vi "(SubVI) path to xy data.vi"(10 "base path":path, 11 "name or relative path":string) -> (1 "all y position\n(pixel)":dbl[][](array[numeric]), 2 "all x position\n(pixel)":dbl[][](array[numeric]), 3 "Tandem Yi position":dbl[](array[numeric]), 4 "# of frames":dbl, 5 "Tandem Xi position":dbl[](array[numeric]), 6 "# of AOIs":dbl)   [LabVIEW 2016]
uses:
  <vilib>/Utility/file.llb/Read Delimited Spreadsheet (string).vi
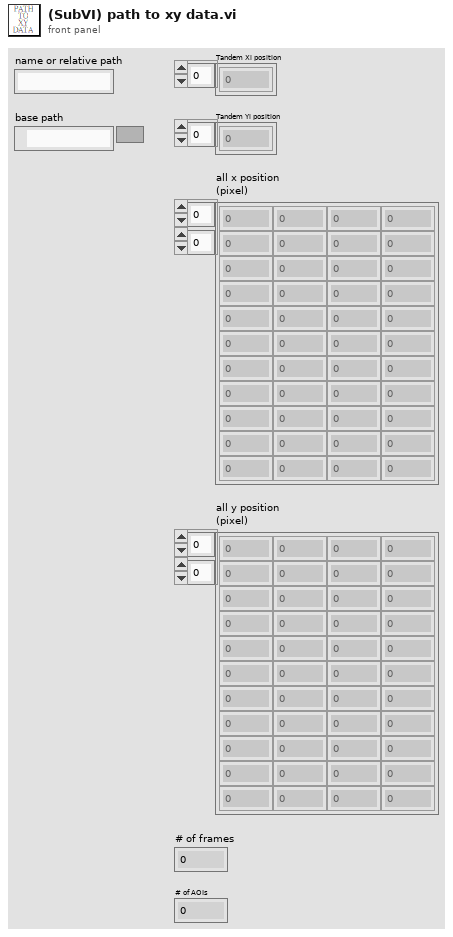
[diagram p1: front panel]
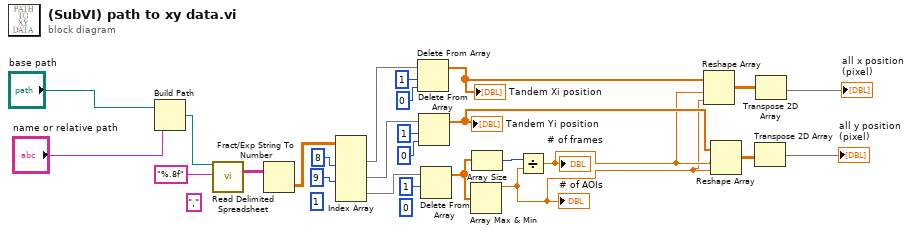
[diagram p0: block diagram]
diagram:
  (unwired) 0 ("index")
  (unwired) 1 ("index (col)")
  (unwired) "," ("delimiter (\\t)")
  n1 = Build Path(base path="base path", name or relative path="name or relative path") -> (appended path=w16:path)
  n2 = call-poly <vilib>:"Read Delimited Spreadsheet.vi"("file path (dialog if empty)"=w16, "format (%s)"="%.8f") -> ("all rows"=w2:string[][])  [unwired: 8 in, 5 out]
  n3 = Fract/Exp String To Number(string=w2) -> (number=w3:dbl[][])  [unwired: 3 in, 1 out]
  n4 = Index Array(array=w3, index (col) #1=8 ("disabled index (col)"), index (col) #2=9 ("index (col)")) -> (element #1=w11:dbl[], element #2=w12:dbl[], element #3=w13:dbl[])  [unwired: 4 in]
  n5 = Delete From Array(array=w11, length=1, index=0) -> (array with subset deleted=w21:dbl[])  [unwired: 1 out]
  "Tandem Xi position" <- w21
  n6 = Delete From Array(array=w12, length=1, index=0) -> (array with subset deleted=w24:dbl[])  [unwired: 1 out]
  "Tandem Yi position" <- w24
  n7 = Delete From Array(array=w13, length=1) -> (array with subset deleted=w14:dbl[])  [unwired: 1 in, 1 out]
  n8 = Array Max & Min(array=w14) -> (max value=w22:dbl)  [unwired: 3 out]
  "# of AOIs" <- w22
  n9 = Array Size(array=w14) -> (size(s)=w15:i32)
  n10 = Divide(x=w15, y=w22) -> (x/y=w23:dbl)
  "# of frames" <- w23
  n11 = Reshape Array(w21, w23, w22) -> (w17:dbl[][])
  n12 = Reshape Array(w24, w23, w22) -> (w18:dbl[][])
  n13 = Transpose 2D Array(2D array=w18) -> (transposed array=→"all y position\n(pixel)":dbl[][])
  n14 = Transpose 2D Array(2D array=w17) -> (transposed array=→"all x position\n(pixel)":dbl[][])
